vi "RF FC limit check.vi"(8 "error in (no error)":errorcluster, 10 "RF Fc":dbl, 11 "reference in":refnum<class "mmWave instrument.lvclass">) -> (0 "error out":errorcluster, 3 "reference out":refnum<class "mmWave instrument.lvclass">)   [LabVIEW 2019, in "mmWave instrument.lvclass"]
doc: "Checks if specified RF value is withing range"
uses:
  mmWave instrument.lvclass
  mmWave HW Control/HW custom error.ctl
  mmWave HW Control/mmWave HW Control.lvlib
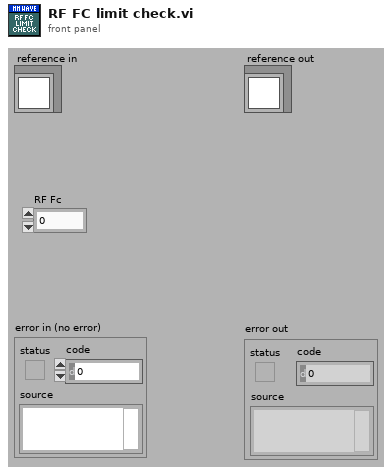
[diagram p1: front panel]
types:
  T1 = typedef "mmWave instrument.lvclass/ObjectAttributes.ctl" = cluster{"mode":T2, "instr state":T3, "Max Fs":dbl, "Equalization coeff":cdb[], "LO sync en":bool, "Trig sync en":bool, "LO sources":T4, "LO Export":T5, "Fc.range":cluster{"min":dbl, "max":dbl}, "Sync mode":T6, "equalization en":bool, "sequence":string[]}
  T2 = typedef "mmWave instrument.lvclass/Instrument mode.ctl" = enum16{"RF", "IF", "BB"}
  T3 = typedef "mmWave instrument.lvclass/Instrument state.ctl" = enum16{"Off", "Initialization", "Configuration", "Running", "Calibration"}
  T4 = typedef "mmWave HW Control.lvlib/LO sources.ctl" = cluster{"RX/LO1 src":string, "TX/LO1 src":string, "LO2 src":string}
  T5 = typedef "mmWave HW Control.lvlib/LO export.ctl" = cluster{"TX LO1 export":bool, "TX LO1 export level":dbl, "RX LO1 export":bool, "RX LO1 export level":dbl, "LO2 export":bool, "LO2 export level":dbl}
  T6 = typedef "mmWave instrument.lvclass/Sync mode.ctl" = enum16{"Slave", "Master"}
  T7 = typedef "mmWave HW Control.lvlib/HW custom error.ctl" = u16
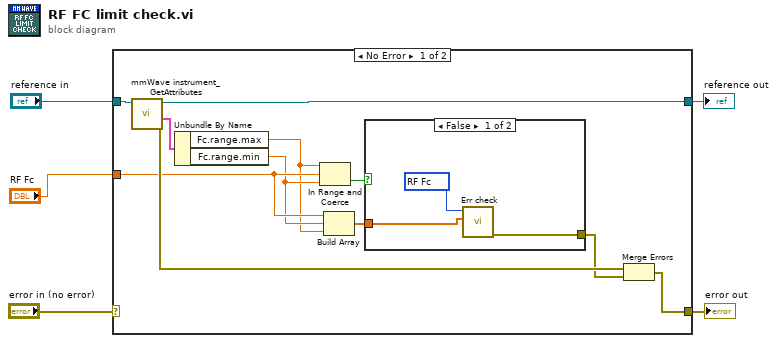
[diagram p0: block diagram]
diagram:
  n1 = case shown="No Error" "error in (no error)" {
    selector: "error in (no error)" -> [_ w21]
    tunnel: [w6 w21] -> w4
    tunnel: [w16 w20] -> w2
    tunnel: "reference in" -> [w14 w20]
    tunnel: "RF Fc" -> [w11 _]
    frame No Error {
      n2 = call "mmWave instrument_GetAttributes.vi"("reference in"=w14) -> ("error out"=w13:errorcluster, "attributes"=w15:T1, "reference out"=w16:refnum<class "mmWave instrument.lvclass">)  [unwired: 7 in, 1 out]
      n3 = Unbundle By Name(w15) -> ("Fc.range.max"=w9:dbl, "Fc.range.min"=w10:dbl)
      n4 = In Range and Coerce(upper limit=w9, x=w11, lower limit=w10) -> (In Range?=w12:bool)  [unwired: 1 out]
      n5 = Build Array(w11, w10, w9) -> (w8:dbl[])
      n6 = case shown="False" w12 {
        tunnel: w8 -> [w19 _]
        tunnel: [w17 _] -> w7
        frame False {
          w18 = T7 10004 items=["TX list"=10000, "TX length"=10001, "RX length"=10002, "Fs"=10003, "RF Fc"=10004] ("HW custom err")
          n7 = call "Err check.vi"("Variant Control"=w19, "HW custom err"=w18) -> ("error out"=w17:errorcluster)  [unwired: 9 in]
        }
        frame True {
        }
      }
      n8 = Merge Errors(w13, w7) -> (w6:errorcluster)
    }
    frame Error {
    }
  }
  "error out" <- w4
  "reference out" <- w2
